vi "Get Tx Generic Frame Payload Map.vi"(8 "error in":errorcluster, 11 "custom device ref in":T1 format="%.0x") -> (0 "error out":errorcluster, 2 "Payload Map":map{string, u8[]}(c390), 3 "custom device ref out":T1 format="%.0x")   [LabVIEW 2020, in "AIM ARINC 664 Scripting.lvlib"]
uses:
  <vilib>/NI VeriStand/Custom Device API/Custom Device Item Ref.ctl
  Constants.vi
  <vilib>/NI VeriStand/Custom Device API/Get Item Property (Variant).vi
  AIM ARINC 664 Scripting.lvlib
  <vilib>/NI VeriStand/Custom Device API/Custom Device API.lvlib
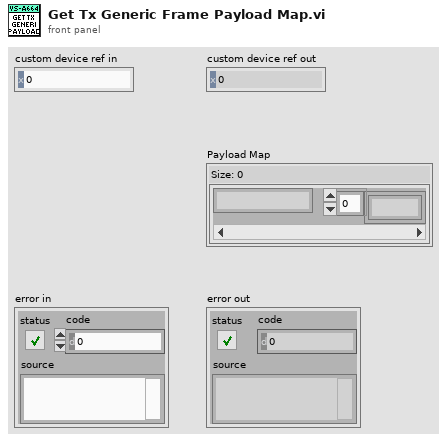
[diagram p1: front panel]
types:
  T1 = typedef "Custom Device API.lvlib/Custom Device Item Ref.ctl" = u64
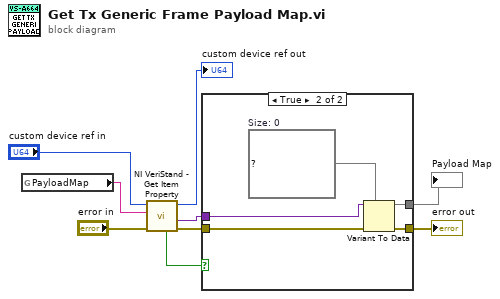
[diagram p0: block diagram]
diagram:
  n1 = global read "Constants.vi" "PayloadMap"() -> (w1:string)
  n2 = call-poly <vilib>:"NI VeriStand - Get Item Property.vi"("error in (no error)"="error in", "Property Name"=w1, "Item Ref in"="custom device ref in") -> ("error out"=w6:errorcluster, "Value"=w4:variant, "Item Ref out"=→"custom device ref out":T1, "Found?"=w5:bool)  [unwired: 5 in]
  n3 = case shown="True" w5 {
    tunnel: w6 -> [w10 w15]
    tunnel: w4 -> [_ w14]
    tunnel: [_ w13] -> w2
    tunnel: [w10 w12] -> w3
    frame False {
    }
    frame True {
      w11 = map{string, u8[]} {}  # Size: 0
      n4 = Variant To Data(error in=w15, type=w11, Variant=w14) -> (data=w13:map{string, u8[]}, error out=w12:errorcluster)
    }
  }
  "error out" <- w3
  "Payload Map" <- w2
